vi "Check Next Trigger State (indexed).vi"(8 "error in (no error)":errorcluster, 10 "Array of States LUT":variant[](array[variant]), 11 "TriggerAction in":refnum<class "TriggerAction Q.lvclass">) -> (0 "error out":errorcluster, 2 "Trigger State":bool, 3 "TriggerAction out":refnum<class "TriggerAction Q.lvclass">)   [LabVIEW 2016, in "TriggerAction Q.lvclass"]
uses:
  <userlib>/Common Components/TriggerAction Q/TriggerAction Q/TriggerAction Q.lvclass
  <userlib>/Common Components/TriggerAction Q/TriggerAction Q/TriggerAction Q.lvclass/TriggerAction Q.ctl
  <userlib>/Common Components/TriggerAction Q/TriggerAction Q/Trigger Cluster.ctl
  <vilib>/Utility/error.llb/Error Cluster From Error Code.vi
  <vilib>/ErrorRing/Error Ring.xnode
  <vilib>/addons/_JKI.lib/Serialization/JSON/JKI JSON Serialization.lvlib
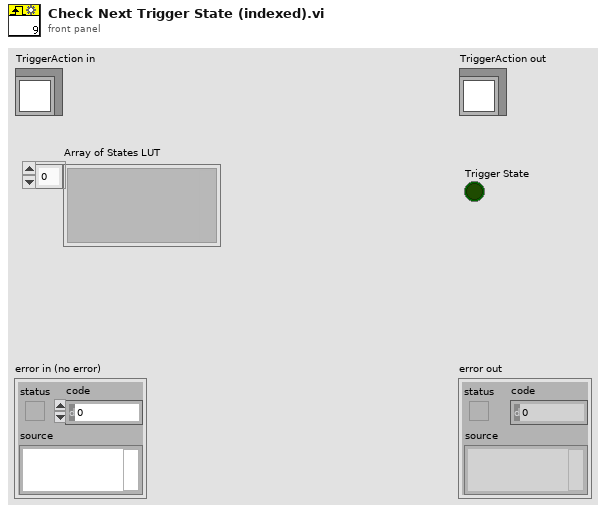
[diagram p1: front panel]
types:
  T1 = typedef "TriggerAction.lvclass/Element Data.ctl" = cluster{"Triggers":cluster{"Triggers for Array AND":string[]}[], "Actions":cluster{"Action Name":string, "Action Data":string}[]}
  T2 = typedef "TriggerAction Q.lvclass/Trigger Cluster.ctl" = cluster{"Index":u8, "State Name":string}
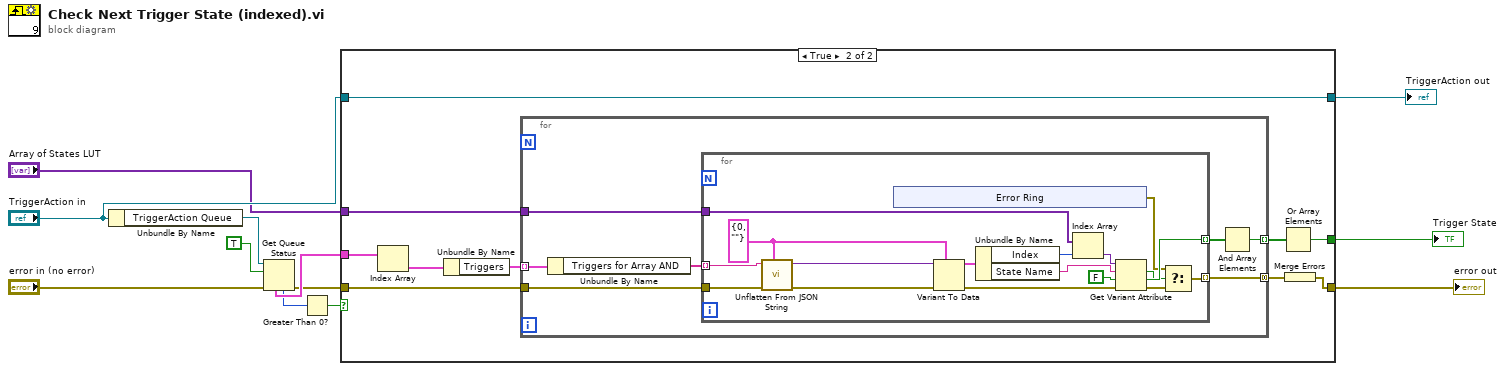
[diagram p0: block diagram]
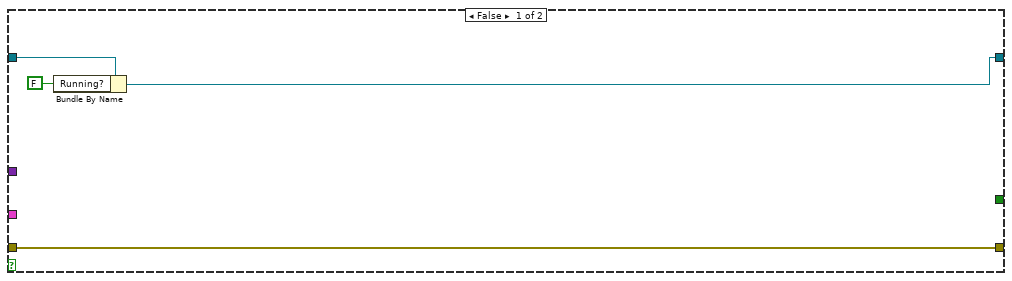
[diagram p2: hidden frame]
diagram:
  n1 = Unbundle By Name("TriggerAction in") -> ("TriggerAction Queue"=w12:refnum<queue>)
  n2 = Get Queue Status(queue=w12, return elements? (F)=TRUE, error in (no error)="error in (no error)") -> (error out=w3:errorcluster, # elements in queue=w8:i32, elements=w10:T1[])  [unwired: 5 out]
  n3 = Greater Than 0?(x=w8) -> (x > 0?=w7:bool)
  n4 = case shown="True" w7 {
    tunnel: w10 -> [_ w26]
    tunnel: "Array of States LUT" -> [_ w23]
    tunnel: [_ w21] -> w9
    tunnel: "TriggerAction in" -> [w16 w20]
    tunnel: [w14 w20] -> w5
    tunnel: w3 -> [w13 w19]
    tunnel: [w13 w17] -> w2
    frame False {
      n5 = Bundle By Name(cluster=w16, "Running?"=FALSE) -> (w14:refnum<class "TriggerAction Q.lvclass">)
    }
    frame True {
      n6 = Index Array(array=w26) -> (element=w25:T1)  [unwired: 1 in]
      n7 = Unbundle By Name(w25) -> ("Triggers"=w24:cluster{"Triggers for Array AND":string[]}[])
      n8 = for {
        tunnel: w24 -> [w32] mode=indexing
        tunnel: w23 -> [w33]
        tunnel: [w29] -> w22 mode=indexing
        tunnel: w19 -> [w28]
        tunnel: [w27] -> w18 mode=concatenating
        n9 = Unbundle By Name(w32) -> ("Triggers for Array AND"=w30:string[])
        n10 = for {
          tunnel: w33 -> [w50]
          tunnel: [w47] -> w31 mode=indexing
          tunnel: w30 -> [w49] mode=indexing
          tunnel: w28 -> [w36]
          tunnel: [w43] -> w27 mode=indexing
          w41 = T2 {"Index"=0, "State Name"=""} ("Cluster")
          n11 = call <vilib>:"Unflatten From JSON String.vi"("Type and Defaults"=w41, "error in (no error)"=w36, "JSON String"=w49) -> ("error out"=w35:errorcluster, "Variant"=w42:variant)  [unwired: 7 in]
          n12 = xnode "Error Ring"() -> ("error out"=w45:errorcluster)
          n13 = Variant To Data(error in=w35, type=w41, Variant=w42) -> (data=w40:T2, error out=w34:errorcluster)
          n14 = Unbundle By Name(w40) -> ("Index"=w38:u8, "State Name"=w37:string)
          n15 = Index Array(array=w50, index=w38) -> (element=w39:variant)
          n16 = Get Variant Attribute(Variant=w39, name=w37, default value (empty Variant)=FALSE, error in=w34) -> (found=w46:bool, value=w47:bool, error out=w44:errorcluster)  [unwired: 1 out]
          n17 = Select(t=w45, s=w46, f=w44) -> (s? t:f=w43:errorcluster)
        }
        n18 = And Array Elements(Boolean array=w31) -> (logical AND=w29:bool)
      }
      n19 = Or Array Elements(Boolean array=w22) -> (logical OR=w21:bool)
      n20 = Merge Errors(w18) -> (w17:errorcluster)
    }
  }
  "error out" <- w2
  "TriggerAction out" <- w5
  "Trigger State" <- w9
